vi "HFRR ADV v10.vi"() -> ()   [LabVIEW 2025] (continued)
                    n4161 = Number To Fractional String(number=w5626, width (-)=i16 10, precision (6)=i16 4) -> (F-format string=w5630:string)  [unwired: 1 in]
                    n4162 = Concatenate Strings("FrictionalForce\":\"", w5630, w5628) -> (w5629:string)
                  }
                  frame #3 {
                    n4163 = local read "Set Hz"() -> (w5634:dbl)
                    n4164 = Multiply(x=w5634, y=60.0) -> (x*y=w5633:dbl)
                    n4165 = Number To Fractional String(number=w5633, width (-)=i16 10, precision (6)=i16 4) -> (F-format string=w5639:string)  [unwired: 1 in]
                    n4166 = Concatenate Strings("Speed\":\"", w5639, w5636) -> (w5638:string)
                  }
                  frame #4 {
                    n4167 = local read "Stroke Ln"() -> (w5642:dbl)
                    n4168 = Number To Fractional String(number=w5642, width (-)=i16 10, precision (6)=i16 4) -> (F-format string=w5646:string)  [unwired: 1 in]
                    n4169 = Concatenate Strings("LinearDeformation\":\"", w5646, w5644) -> (w5643:string)
                  }
                  frame #5 {
                    n4170 = local read "AIR TEMP"() -> (w5649:dbl)
                    n4171 = local read "Json St Flg"() -> (w5651:bool)
                    n4172 = local read "Json End Flg"() -> (w5652:bool)
                    n4173 = Number To Fractional String(number=w5649, width (-)=i16 10, precision (6)=i16 4) -> (F-format string=w5655:string)  [unwired: 1 in]
                    n4174 = Concatenate Strings("Vibration\":\"", w5655, w5653) -> (w5650:string)
                    n4175 = And(x=w5651, y=w5652) -> ()  [unwired: 1 out]
                  }
                  frame #6 {
                    n4176 = local read "Json End Flg"() -> (w5659:bool)
                    n4177 = Get Date/Time In Seconds() -> (seconds since 1Jan1904=w5667:timestamp)
                    n4178 = local read "Json St Flg"() -> (w5658:bool)
                    n4179 = To Double Precision Float(number=w5667) -> (double precision float=w5666:dbl)
                    n4180 = Subtract(x=w5666, y=2082844800.0) -> (x-y=w5664:dbl)
                    n4181 = Number To Fractional String(number=w5664, width (-)=i16 12, precision (6)=i16 0) -> (F-format string=w5661:string)  [unwired: 1 in]
                    n4182 = case shown="True" w5659 {
                      tunnel: ["" w5674] -> w5668
                      tunnel: w5661 -> [_ w5675]
                      tunnel: w5660 -> [_ w5673]
                      frame False {
                      }
                      frame True {
                        n4183 = local write "Json End Flg"(FALSE ("Json St Flg")) -> ()
                        n4184 = Concatenate Strings("End\": \"", w5675, w5673) -> (w5674:string)
                      }
                    }
                    n4185 = case shown="True" w5658 {
                      tunnel: [w5678 w5681] -> w5669
                      tunnel: w5661 -> [_ w5682]
                      tunnel: w5660 -> [_ w5679]
                      frame False {
                        n4186 = local read "St Str"() -> (w5678:string)
                      }
                      frame True {
                        n4187 = Concatenate Strings("Start\":\"", w5682, w5679) -> (w5681:string)
                        "St Str" <- w5681
                        n4188 = local write "Json St Flg"(FALSE ("Json St Flg")) -> ()
                      }
                    }
                    n4189 = Concatenate Strings(w5669, w5668, w5671) -> (w5670:string)
                  }
                }
                n4190 = local read "FILE"() -> (w5539:string)
                n4191 = Concatenate Strings("\",\"OperatorID\":\"" ("string"), "Operator ID") -> (w5542:string)
                n4192 = Concatenate Strings("\",\"DatasetTitle\":\"" ("string"), w5539) -> (w5541:string)
                n4193 = Concatenate Strings("\",\"SerialNumber\":\"" ("string"), "Serial No") -> (w5571:string)
                n4194 = Concatenate Strings("\",\"ModelNumber\":\"" ("string"), "Model No") -> (w5570:string)
                n4195 = Concatenate Strings(w5571, w5570) -> (w5553:string)
                n4196 = Concatenate Strings("{\"SecretKey\":\"", "Secret Key", w5553, w5542, w5541, "\",\"Samples\":[") -> (w5558:string)
                n4197 = Concatenate Strings(w5560, w5564, w5563, w5562, w5561, w5545, w5546, w5547) -> (w5559:string)
                n4198 = Concatenate Strings(w5558, w5559, "]}") -> (w5557:string)
                n4199 = stacked-sequence {
                  tunnel: w5557 -> [w5586 _ _]
                  tunnel: [_ _ w5603] -> _
                  frame #0 {
                    (unwired) FALSE ("convert eol (F)")
                    w5588 = enum16{"start", "end", "current"}."start" ("pos mode (0:2)")
                    n4200 = Path To String(path="Path") -> (string=w5594:string)
                    n4201 = Concatenate Strings(w5594, "\\", "Data File Name") -> (w5596:string)
                    n4202 = local write "standard output"(" ") -> ()
                    n4203 = String To Path(string=w5596) -> (path=w5585:path)
                    n4204 = call <vilib>:"Open_Create_Replace File.vi"("advisory dialog? (display:T)"=FALSE, "function (open:0)"=T28."create or replace", "file path"=w5585) -> ("error out"=w5599:errorcluster, "refnum"=w5598:refnum<file>)  [unwired: 5 in, 2 out]
                    n4205 = Set File Position(refnum=w5598, from (0:start)=w5588, error in=w5599) -> (refnum out=w5579:refnum<file>, error out=w5578:errorcluster)  [unwired: 1 in]
                    n4206 = Write to Binary File(file (use dialog)=w5579, data=" ", error in=w5578, 5:FALSE ("prepend array or string size? (T)")) -> (refnum out=w5589:refnum<file>, error out=w5590:errorcluster)  [unwired: 2 in, 1 out]
                    n4207 = Set File Position(offset (in bytes) (0)=w5588, refnum=w5589, error in=w5590) -> (refnum out=w5582:refnum<file>, error out=w5581:errorcluster)  [unwired: 1 in]
                    n4208 = Write to Binary File(file (use dialog)=w5582, data=w5586, error in=w5581, 5:FALSE ("prepend array or string size? (T)")) -> (error out=w5584:errorcluster)  [unwired: 2 in, 2 out]
                    n4209 = flat-sequence {
                      tunnel: w5585 -> [w5601]
                      tunnel: w5584 -> [_]
                      frame #0 {
                        n4210 = call <vilib>:"Read Characters From File.vi"("file path (dialog if empty)"=w5601) -> ("character string"=→"JSON string":string)  [unwired: 5 in, 3 out]
                      }
                    }
                    "SinglePoint" <- w5586
                  }
                  frame #1 {
                  }
                  frame #2 {
                    (unwired) "\"Stored\": true" ("string")
                    n4211 = call <vilib>:"System Exec.vi"("run minimized? (F)"=TRUE, "wait until completion? (T)"=TRUE, "working directory"=path "C:/LAB-IQ-NXT", "command line"="C:\\LAB-IQ-NXT\\JPost.bat") -> ("standard error"=→"Respose From Server":string, "standard output"=w5606:string)  [unwired: 4 in, 2 out]
                    "standard output" <- w5606
                    n4212 = Match Pattern(string=w5606, regular expression="JSON Check String") -> (match substring=w5604:string, offset past match=w5603:i32)  [unwired: 1 in, 2 out]
                    n4213 = Equal?(x=w5604, y="JSON Check String") -> (x = y?=→"Upload \nConfirmed":bool)
                  }
                }
              }
            }
            n4214 = local read "Quit"() -> (w5527:bool)
          }
        }
      }
    }
    frame Enabled {
    }
  }
  n4215 = disable-structure shown="Disabled" {
    disable-tunnel: _ -> [w5689 _]
    frame Disabled {
      n4216 = while {
        shift-right: [w5697] -> w5685
        shift-left: _ -> [w5698]
        shift-right: [w5695] -> w5686
        shift-left: errorcluster {"status"=TRUE, "code"=0, "source"="Init"} ("error out") -> [w5696]
        shift-right: [w5693] -> _
        shift-left: "" -> [w5694]
        tunnel: [w5691] -> _
        tunnel: w5689 -> [_]
        i -> [w5691]
        stop <- w5690 stop-if-true
        n4217 = flat-sequence {
          tunnel: [w5699] -> w5692
          frame #0 {
            n4218 = Wait (ms)(milliseconds to wait=10.0 ("Delay")) -> (millisecond timer value=w5699:u32)
          }
        }
        n4219 = case shown="No Error" w5696 {
          selector: w5696 -> [w5732 w5854]
          tunnel: [w5714 w5856] -> w5697
          tunnel: [w5713 w5855] -> w5695
          tunnel: w5698 -> [w5733 w5848]
          tunnel: w5694 -> [w5712 w5847]
          tunnel: [w5711 w5847] -> w5693
          tunnel: w5692 -> [_ _]
          frame No Error {
            n4220 = Concatenate Strings("COMMAND", "\r", "\n") -> (w5723:string)
            n4221 = case shown="True" "Measure" {
              tunnel: w5733 -> [w5759 w5766]
              tunnel: w5732 -> [w5758 w5765]
              tunnel: [w5759 w5764] -> w5731
              tunnel: [w5758 w5763] -> w5710
              tunnel: w5723 -> [_ w5762]
              frame False {
              }
              frame True {
                n4222 = VISA Write(VISA resource name=w5766, write buffer=w5762, error in (no error)=w5765) -> (VISA resource name out=w5764:refnum<visa-resource-name>, error out=w5763:errorcluster)  [unwired: 1 out]
                n4223 = local write "Read String"("") -> ()
                n4224 = local write "Measure"(FALSE) -> ()
              }
            }
            n4225 = property class="Instr"(reference=w5731, error in=w5710) -> (reference out=w5730:refnum<visa-resource-name>, error out=w5729:errorcluster, "Serial Settings:Number of Bytes at Serial Port"=w5728:u32)
            n4226 = Greater?(x=w5728, y=u32 100) -> (0:w5726:bool)
            n4227 = case shown="True" w5726 {
              tunnel: w5730 -> [w5769 w5794]
              tunnel: w5729 -> [w5768 w5793]
              tunnel: w5728 -> [_ w5792]
              tunnel: [w5769 w5791] -> w5716
              tunnel: [w5768 w5790] -> w5715
              tunnel: w5712 -> [w5767 w5789]
              tunnel: [w5767 ""] -> w5711
              frame False {
              }
              frame True {
                w5779 = u32 6 ("y")
                # "Page 84 of \nmanual"
                n4228 = VISA Read(VISA resource name=w5794, byte count=w5792, error in (no error)=w5793) -> (VISA resource name out=w5791:refnum<visa-resource-name>, read buffer=w5787:string, error out=w5790:errorcluster)  [unwired: 1 out]
                n4229 = while {
                  tunnel: w5787 -> [w5843]
                  tunnel: [w5839] -> w5781 mode=indexing
                  tunnel: [w5833] -> w5785 mode=indexing
                  tunnel: [w5831] -> _
                  i -> [w5831]
                  stop <- w5836 stop-if-true
                  n4230 = String Subset(string=w5843, offset (0)=w5831) -> (substring=w5838:string)  [unwired: 1 in]
                  n4231 = String To Byte Array(string=w5838) -> (unsigned byte array=w5842:u8[])
                  n4232 = String Length(string=w5838) -> (length=w5837:i32)
                  n4233 = Index Array(array=w5842) -> (element=w5841:u8)  [unwired: 1 in]
                  n4234 = Equal To 0?(x=w5837) -> (x = 0?=w5836:bool)
                  n4235 = Number To Boolean Array(number=w5841) -> (Boolean array=w5835:bool[])
                  n4236 = Reverse 1D Array(array=w5835) -> (reversed array=w5834:bool[])
                  n4237 = And(x=w5835, y=bool[] [FALSE, FALSE, FALSE, FALSE, FALSE, FALSE, TRUE, TRUE] ("Boolean array")) -> (x .and. y?=w5839:bool[])
                  n4238 = And(x=w5834, y=bool[] [FALSE, FALSE, TRUE, TRUE, TRUE, TRUE, TRUE, TRUE] ("Boolean array")) -> (x .and. y?=w5833:bool[])
                }
                n4239 = Concatenate Strings(w5789, w5787) -> (→"Read String":string)
                n4240 = while {
                  tunnel: w5781 -> [w5830] mode=indexing
                  tunnel: [w5826] -> w5784
                  i -> [w5826]
                  stop <- w5827 stop-if-true
                  n4241 = Search 1D Array(1D array=w5830, element=TRUE) -> (index of element=w5828:i32)  [unwired: 1 in]
                  n4242 = Less Than 0?(x=w5828) -> (x < 0?=w5827:bool)
                }
                n4243 = Delete From Array(array=w5785, length=w5784, index (row)=0) -> (array with subset deleted=w5780:bool[][])  [unwired: 1 in, 1 out]
                n4244 = Array Size(array=w5780) -> (size(s)=w5782:i32[])
                n4245 = Index Array(array=w5782) -> (element=w5774:i32)  [unwired: 1 in]
                n4246 = Greater?(x=w5774, y=w5779) -> (0:w5777:bool)
                n4247 = Subtract(x=w5774, y=w5779) -> (x-y=w5778:u32)
                n4248 = Select(t=w5778, s=w5777, f=u32 0) -> (s? t:f=w5775:u32)
                n4249 = while {
                  tunnel: w5780 -> [w5813]
                  tunnel: [w5815] -> w5773 mode=indexing
                  tunnel: w5775 -> [w5797]
                  i -> [w5814]
                  stop <- w5812 stop-if-true
                  w5804 = 6 ("index")
                  w5803 = 2 ("length")
                  # "Page 65 of \nmanual"
                  n4250 = Multiply(x=u32 3 ("y"), y=w5814) -> (x*y=w5811:u32)
                  n4251 = Divide(x=u32 102 ("y"), y=u32 65520) -> (x/y=w5821:dbl)
                  n4252 = Greater Or Equal?(x=w5811, y=w5797) -> (x >= y?=w5812:bool)
                  n4253 = Index Array(array=w5813, index (row) #1=w5811) -> (element #1=w5809:bool[], element #2=w5808:bool[], element #3=w5807:bool[])  [unwired: 5 in]
                  n4254 = Reverse 1D Array(array=w5809) -> (reversed array=w5802:bool[])
                  n4255 = Reverse 1D Array(array=w5808) -> (reversed array=w5806:bool[])
                  n4256 = Reverse 1D Array(array=w5807) -> (reversed array=w5805:bool[])
                  n4257 = Delete From Array(array=w5802, length=w5803, index=w5804) -> (array with subset deleted=w5798:bool[])  [unwired: 1 out]
                  n4258 = Delete From Array(array=w5806, length=w5803, index=w5804) -> (array with subset deleted=w5799:bool[])  [unwired: 1 out]
                  n4259 = Delete From Array(array=w5805, length=w5803, index=w5804) -> (array with subset deleted=w5800:bool[])  [unwired: 1 out]
                  n4260 = Insert Into Array(array=bool[] [] ("Boolean array"), new element #1=w5798, new element #2=w5799, new element #3=w5800) -> (w5801:bool[])  [unwired: 1 in]
                  n4261 = Boolean Array To Number(Boolean array=w5801) -> (number=w5810:u32)
                  n4262 = Multiply(x=w5821, y=w5810) -> (x*y=w5820:dbl)
                  n4263 = Decrement(x=w5820) -> (x-1=w5819:dbl)
                  n4264 = Divide(x=w5819, y=u32 100) -> (x/y=w5817:dbl)
                  n4265 = Multiply(x=w5817, y=u32 10) -> (x*y=w5815:dbl)
                }
                n4266 = Delete From Array(array=w5773) -> (array with subset deleted=w5772:dbl[])  [unwired: 2 in, 1 out]
                "Waveform Graph 5" <- w5772
                "Waveform Chart 3" <- w5772
                n4267 = call-poly <vilib>:"Mean.vi"("X"=w5772) -> ("mean"=w5771:dbl)  [unwired: 1 out]
                "Measure_LDS" <- w5771
                n4268 = case shown="True" "Zero 4" {
                  tunnel: w5771 -> [_ w5796]
                  frame False {
                  }
                  frame True {
                    n4269 = local write "Zero 4"(FALSE ("Zero 4")) -> ()
                    "z_measure" <- w5796
                  }
                }
              }
            }
            n4270 = local read "Measure_LDS"() -> (w5706:dbl)
            n4271 = local read "Disp (mm)"() -> (w5705:dbl)
            n4272 = local read "Boolean 7"() -> (w5704:bool)
            n4273 = local read "Boolean 8"() -> (w5703:bool)
            n4274 = case shown="True" "Boolean 8" {
              tunnel: w5705 -> [_ w5736]
              tunnel: w5706 -> [_ w5735]
              frame False {
              }
              frame True {
                n4275 = local read "Captured Values 2"() -> (w5739:dbl[][])
                n4276 = Build Array(w5736, w5735) -> (w5734:dbl[])
                n4277 = Build Array (concatenate)(w5739, w5734) -> (w5737:dbl[][])
                n4278 = local write "Captured Values 2"(w5737) -> ()
                n4279 = local write "Boolean 8"(FALSE ("Boolean 8")) -> ()
              }
            }
            n4280 = call "Build XY Graph"("Enable"=w5703, "Reset"=w5704, "Y Input"=w5706, "X Input"=w5705) -> ("XY Graph"=→"?":cluster{"Y":dbl[], "Y":dbl[]}[])  [unwired: 6 in, 1 out]
            n4281 = case shown="True" "Boolean 9" {
              frame False {
              }
              frame True {
                n4282 = local read "Captured Values 2"() -> (w5741:dbl[][])
                n4283 = Index Array(array=w5741, index (col) #1=0 ("disabled index (col)"), index (col) #2=1 ("index (col)")) -> (element #1=w5744:dbl[], element #2=w5743:dbl[])  [unwired: 2 in]
                n4284 = call <vilib>:"Linear Fit.vi"("Y"=w5744, "X"=w5743) -> ("slope"=→"Slope":dbl, "intercept"=→"Intercept":dbl)  [unwired: 9 in, 3 out]
                n4285 = local write "Boolean 9"(FALSE ("Boolean 9")) -> ()
              }
            }
            n4286 = case shown="True" "Boolean 7" {
              frame False {
              }
              frame True {
                n4287 = local write "Captured Values 2"(dbl[][] [] ("Captured Values")) -> ()
                n4288 = local write "Boolean 7"(FALSE ("Boolean 7")) -> ()
              }
            }
            n4289 = Concatenate Strings("COMMAND 2", "\r", "\n") -> (w5718:string)
            n4290 = case shown="True" "Measure 2" {
              tunnel: w5716 -> [w5751 w5757]
              tunnel: w5715 -> [w5750 w5756]
              tunnel: [w5751 w5755] -> w5714
              tunnel: [w5750 w5754] -> w5713
              tunnel: w5718 -> [_ w5753]
              frame False {
              }
              frame True {
                n4291 = local write "Measure 2"(FALSE ("WRITE")) -> ()
                n4292 = VISA Write(VISA resource name=w5757, write buffer=w5753, error in (no error)=w5756) -> (VISA resource name out=w5755:refnum<visa-resource-name>, error out=w5754:errorcluster)  [unwired: 1 out]
              }
            }
          }
          frame Error {
            w5846 = u16 10 items=["1.0"=10, "1.5"=15, "2.0"=20] ("stop bits (10: 1 bit)")
            n4293 = Wait (ms)(milliseconds to wait=u32 20) -> ()  [unwired: 1 out]
            n4294 = VISA Close(VISA resource name=w5848, error in (no error)=w5854) -> (error out=w5853:errorcluster)
            n4295 = call <vilib>:"Clear Errors.vi"("error in (no error)"=w5853) -> ("error out"=w5852:errorcluster)  [unwired: 5 in, 1 out]
            n4296 = call-poly "VISA Configure Serial Port"("VISA resource name"="Laser Disp Sensor", "timeout (10sec)"=u32 200, "Enable Termination\nChar (T)"=TRUE ("Enable Termination\nChar (T)"), "baud rate (9600)"=u32 921600, "error in (no error)"=w5852, "stop bits (10: 1 bit)"=w5846) -> ("VISA resource name out"=w5856:refnum<visa-resource-name>, "error out"=w5855:errorcluster)  [unwired: 8 in]
          }
        }
        n4297 = local read "Quit"() -> (w5690:bool)
      }
      n4298 = VISA Close(VISA resource name=w5685, error in (no error)=w5686) -> (error out=w5684:errorcluster)
      n4299 = call <vilib>:"Clear Errors.vi"("error in (no error)"=w5684) -> ()  [unwired: 5 in, 2 out]
    }
    frame Enabled {
    }
  }
  n4300 = disable-structure shown="Disabled" {
    disable-tunnel: _ -> [w5861 _]
    frame Disabled {
      n4301 = while {
        tunnel: [w5868] -> _
        shift-right: [w5865] -> w5858
        shift-left: _ -> [w5867]
        shift-right: [w5866] -> w5859
        shift-left: errorcluster {"status"=TRUE, "code"=0, "source"="Init"} ("error out") -> [w5864]
        tunnel: w5861 -> [_]
        i -> [w5868]
        stop <- w5862 stop-if-true
        n4302 = flat-sequence {
          tunnel: w5864 -> [w5959]
          tunnel: [w5959] -> w5863
          frame #0 {
            n4303 = Wait (ms)(milliseconds to wait=u32 50) -> ()  [unwired: 1 out]
          }
        }
        n4304 = case shown="No Error" w5863 {
          selector: w5863 -> [w5909 w5952]
          tunnel: w5867 -> [w5908 w5951]
          tunnel: [w5875 w5942] -> w5866
          tunnel: [w5876 w5950] -> w5865
          frame No Error {
            w5902 = T29 {"Mode"=enum."RTU", "Slave Address"=1} ("Serial Parameters")
            n4305 = call-poly <vilib>:"MB Serial Master Query (poly).vi"("VISA resource name"=w5908, "Starting Address"=i16 1000, "Quantity"=u16 1, "Timeout"=u32 1000, "error in"=w5909, "Serial Parameters"=w5902) -> ("VISA resource name out"=w5903:refnum<visa-resource-name>, "Input Registers"=w5905:u16[], "error out"=w5901:errorcluster)  [unwired: 10 in, 1 out]
            n4306 = Random Number (0-1)() -> (number: 0 to 1=w5890:dbl)
            n4307 = Index Array(array=w5905, index=0) -> (element=w5900:u16)
            n4308 = Subtract(x=w5890, y=0.5) -> (x-y=w5889:dbl)
            n4309 = Divide(x=w5900, y=10 ("index")) -> (x/y=w5894:dbl)
            n4310 = Multiply(x=w5889, y=0.5) -> (x*y=w5888:dbl)
            n4311 = Add(x=w5894, y=w5888) -> (x+y=w5893:dbl)
            n4312 = local read "Amb temp"() -> (w5877:dbl)
            n4313 = Multiply(x=w5893, y=0.2) -> (x*y=w5897:dbl)
            n4314 = Multiply(x=w5877, y=0.8) -> (x*y=w5895:dbl)
            n4315 = Add(x=w5897, y=w5895) -> (x+y=w5878:dbl)
            n4316 = local read "set temp old"() -> (w5872:dbl)
            n4317 = local write "Amb temp"(w5878) -> ()
            n4318 = Select(t="SetTemp 2", s="Heater", f=100.0) -> (s? t:f=w5873:dbl)
            n4319 = Not Equal?(x=w5873, y=w5872) -> (x != y?=w5871:bool)
            n4320 = case shown="True" w5871 {
              tunnel: w5903 -> [w5937 w5939]
              tunnel: [w5936 w5939] -> w5883
              tunnel: w5901 -> [w5935 w5938]
              tunnel: [w5934 w5938] -> w5881
              tunnel: w5873 -> [w5929 _]
              tunnel: w5902 -> [w5931 w5940]
              tunnel: [w5931 w5940] -> w5884
              frame True {
                n4321 = Multiply(x=w5929, y=10 ("index")) -> (x*y=w5928:dbl)
                n4322 = call-poly <vilib>:"MB Serial Master Query (poly).vi"("VISA resource name"=w5937, "Address"=u16 0, "Holding Register"=w5928, "Timeout"=u32 1000, "error in"=w5935, "Serial Parameters"=w5931) -> ("VISA resource name out"=w5936:refnum<visa-resource-name>, "error out"=w5934:errorcluster)  [unwired: 11 in, 1 out]
                "set temp old" <- w5929
              }
              frame False {
              }
            }
            n4323 = flat-sequence {
              tunnel: [w5910] -> _
              tunnel: [w5910] -> w5880
              tunnel: w5881 -> [w5910]
              frame #0 {
                n4324 = Wait (ms)(milliseconds to wait=u32 100) -> ()  [unwired: 1 out]
              }
            }
            n4325 = call "Elapsed Time12"("Time Target (s)"=2.0, "Auto Reset"=TRUE) -> ("Time has Elapsed"=w5885:bool)  [unwired: 10 in, 7 out]
            n4326 = case shown="True" w5885 {
              tunnel: w5884 -> [w5914 w5927]
              tunnel: [w5914 w5927] -> _
              tunnel: [w5913 w5925] -> w5876
              tunnel: w5883 -> [w5913 w5926]
              tunnel: [w5912 w5923] -> w5875
              tunnel: w5880 -> [w5912 w5924]
              frame False {
              }
              frame True {
                n4327 = call-poly <vilib>:"MB Serial Master Query (poly).vi"("VISA resource name"=w5926, "Starting Address"=i16 1003 ("Addr"), "Quantity"=u16 1, "Timeout"=u32 1000, "error in"=w5924, "Serial Parameters"=w5927) -> ("VISA resource name out"=w5925:refnum<visa-resource-name>, "Input Registers"=w5920:u16[], "error out"=w5923:errorcluster)  [unwired: 10 in, 1 out]
                n4328 = Index Array(array=w5920, index=0) -> (element=w5919:u16)
                n4329 = Divide(x=w5919, y=u16 10) -> (x/y=w5915:dbl)
                n4330 = local write "set temp old"(w5915) -> ()
                n4331 = local write "SetTemp"(w5915) -> ()
              }
            }
            "Error Code" <- w5875
            n4332 = Unbundle(w5875) -> ("status"=→"TK4 status":bool)  [unwired: 2 out]
            "SetTemp" <- "SetTemp 2"
          }
          frame Error {
            w5954 = u16 0 items=["None", "Odd", "Even", "Mark", "Space"] ("Parity")
            w5955 = u16 0 items=["None", "XON/XOFF", "RTS/CTS", "XON/XOFF & RTS/CTS", "DTR/DSR", "XON/XOFF & DTR/DSR"] ("Flow Control")
            n4333 = VISA Clear(VISA resource name=w5951, error in (no error)=w5952) -> (VISA resource name out=w5945:refnum<visa-resource-name>, error out=w5943:errorcluster)
            n4334 = VISA Close(VISA resource name=w5945, error in (no error)=w5943) -> (error out=w5944:errorcluster)
            n4335 = call <vilib>:"Clear Errors.vi"("error in (no error)"=w5944) -> ("error out"=w5953:errorcluster)  [unwired: 5 in, 1 out]
            n4336 = Unbundle By Name(T29 {"Mode"=enum."RTU", "Slave Address"=1} ("input cluster")) -> ("Mode"=w5956:enum16{"RTU", "ASCII"})
            n4337 = call <vilib>:"MB Serial Init.vi"("Timeout"=u32 100, "Flow Control"=w5955, "Mode"=w5956, "error in (no error)"=w5953, "Parity"=w5954, "Baud Rate"=u32 9600, "VISA resource name"="Lubrication System COM Port :") -> ("error out"=w5942:errorcluster, "VISA resource name out"=w5950:refnum<visa-resource-name>)  [unwired: 3 in]
            n4338 = local write "set temp old"(0.0 ("set temp old")) -> ()
            n4339 = Unbundle(w5942) -> ("status"=w5941:bool)  [unwired: 2 out]
            n4340 = case shown="True" w5941 {
              selector: w5941 -> [_ w5958]
              frame False {
              }
              frame True {
                n4341 = local write "TK4 status"(w5958) -> ()
              }
            }
          }
        }
        n4342 = local read "Quit"() -> (w5862:bool)
      }
      n4343 = VISA Close(VISA resource name=w5858, error in (no error)=w5859) -> (error out=w5857:errorcluster)
      n4344 = call <vilib>:"Clear Errors.vi"("error in (no error)"=w5857) -> ()  [unwired: 5 in, 2 out]
    }
    frame Enabled {
    }
  }
  "file count" <- 0 ("file count")
